vi "CameraSetup.vi"(3 "error in":errorcluster, 4 "Image Type":T1 items=["Grayscale (U8)", "Grayscale (I16)", "Grayscale (SGL)", "Complex (CSG)", "RGB (U32)", "HSL (U32)", "RGB (U64)", "Grayscale (U16)"], 5 "Camera Name":T2="cam0", 6 "Video Modes":i32(listbox)=20) -> (0 "error out":errorcluster, 1 "New Image":T3, 2 "Session Out":T2)   [LabVIEW 2009]
uses:
  <vilib>/userDefined/High Color/IMAQdx.ctl
  <vilib>/vision/Image Controls.llb/IMAQ Image.ctl
  <vilib>/vision/driver/NI_Vision_Acquisition_Software.lvlib
  Program Files/National Instruments/LabVIEW 2009/resource/objmgr/imaqdx.rc
  <vilib>/vision/NI_Vision_Development_Module.lvlib
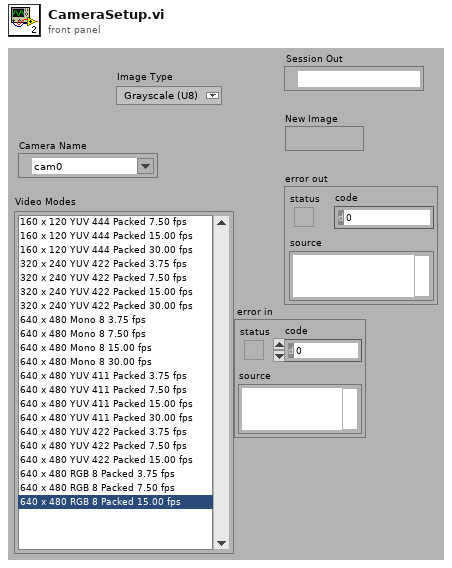
[diagram p1: front panel]
types:
  T1 = typedef "Image Type" = u32
  T2 = typedef "IMAQdx.ctl" = refnum<k21>
  T3 = typedef "IMAQ Image.ctl" = refnum<image>
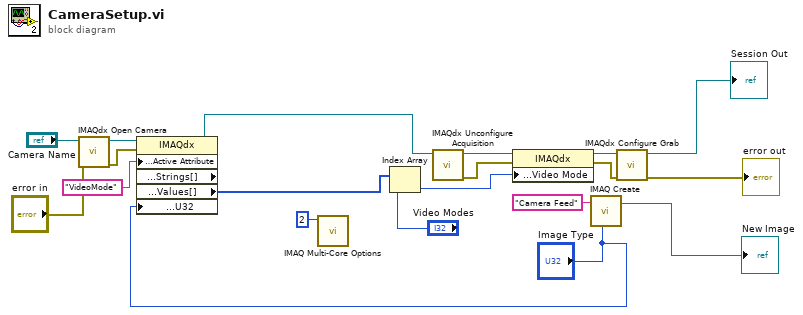
[diagram p0: block diagram]
diagram:
  n1 = call <vilib>:"IMAQdx Open Camera.vi"("error in"="error in", "Session In"="Camera Name") -> ("error out"=w4:errorcluster, "Session Out"=w6:T2)  [unwired: 1 in, 7 out]
  n2 = property class="IMAQdx" props=["Camera Attributes:Active Attribute", "Camera Attributes:Enum:Strings[]", "Camera Attributes:Enum:Values[]", "Camera Attributes:Value:U32"](reference=w6, error in=w4, "Camera Attributes:Active Attribute"="VideoMode" ("ActiveAttribute"), "Camera Attributes:Value:U32"="Image Type") -> (reference out=w15:T2, "Camera Attributes:Enum:Values[]"=w16:u32[])  [unwired: 2 out]
  n3 = call "IMAQ Multi-Core Options"("Specified Number of Cores"=u32 2) -> ()  [unwired: 9 in, 2 out]
  n4 = Index Array(array=w16, index="Video Modes") -> (element=w13:u32)
  n5 = call <vilib>:"IMAQdx Unconfigure Acquisition.vi"("Session In"=w15) -> ("error out"=w12:errorcluster, "Session Out"=w9:T2)  [unwired: 1 in, 8 out]
  n6 = property class="IMAQdx"(reference=w9, error in=w12, "Acquisition Attributes:Video Mode"=w13) -> (reference out=w10:T2, error out=w11:errorcluster)
  n7 = call "IMAQ Create"("Image Name"="Camera Feed", "Image Type"="Image Type") -> ("New Image"=→"New Image":T3)  [unwired: 2 in, 2 out]
  n8 = call <vilib>:"IMAQdx Configure Grab.vi"("error in"=w11, "Session In"=w10) -> ("error out"=→"error out":errorcluster, "Session Out"=→"Session Out":T2)  [unwired: 1 in, 7 out]
